vi "Default.vi"(6 "error in":errorcluster, 9 "Control Terminal in":refnum<class "ControlTerminal.lvclass">) -> (0 "error out":errorcluster, 3 "Control Terminal out":refnum<class "ControlTerminal.lvclass">, 4 "default":string)   [LabVIEW 2014, in "Raspberry Pi Compatible Compiler for LabVIEW.lvlib" / "ControlTerminal.lvclass"]
uses:
  ControlTerminal.lvclass
  Python/Parsing/Python Functions.lvlib
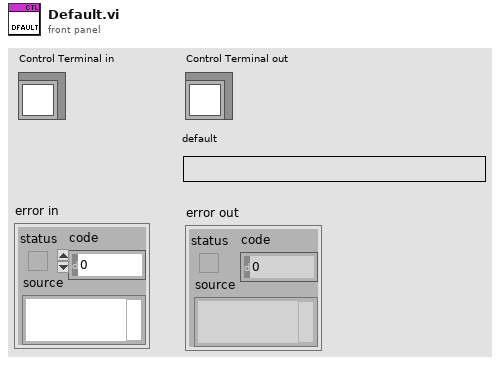
[diagram p1: front panel]
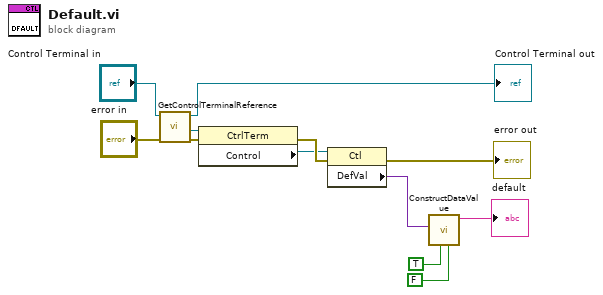
[diagram p0: block diagram]
diagram:
  n1 = call "GetControlTerminalReference.vi"("error in"="error in", "ControlTerminal in"="Control Terminal in") -> ("error out"=w6:errorcluster, "reference"=w5:refnum<vi>, "ControlTerminal out"=→"Control Terminal out":refnum<class "ControlTerminal.lvclass">)  [unwired: 7 in]
  n2 = property class="CtrlTerm"(reference=w5, error in=w6) -> (error out=w10:errorcluster, "Control"=w9:refnum<vi>)  [unwired: 1 out]
  n3 = property class="Ctl"(reference=w9, error in=w10) -> (error out=→"error out":errorcluster, "DefVal"=w12:variant)  [unwired: 1 out]
  n4 = call "ConstructDataValue.vi"("label"=FALSE, "value"=TRUE, "Value"=w12) -> ("value"=→"default":string)  [unwired: 5 in, 1 out]
